vi "Rotation.vi"(8 "C Y":dbl=540.0, 9 "C X":dbl=960.0, 10 "Y":dbl, 11 "X":dbl) -> (1 "Rot Y":dbl, 2 "Rot X":dbl)   [LabVIEW 2020, in "obs-scratch.lvlib"]
uses:
  obs-scratch.lvlib
panel:
  in  "Rotation":dbl(slide) scale=-180.0..180.0
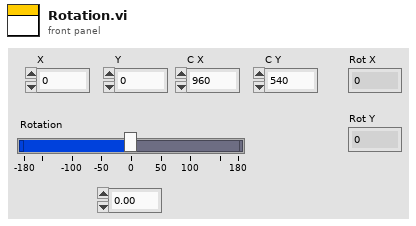
[diagram p1: front panel]
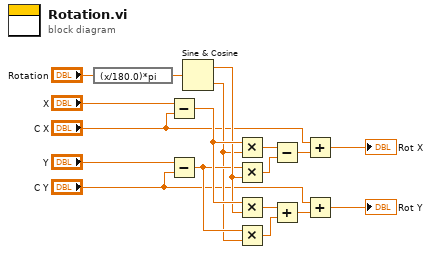
[diagram p0: block diagram]
diagram:
  n1 = expression code="(x/180.0)*pi" ("degrees to radians")("Rotation") -> (w7:dbl)
  n2 = Subtract(x="X", y="C X") -> (x-y=w13:dbl)
  n3 = Subtract(x="Y", y="C Y") -> (x-y=w11:dbl)
  n4 = Sine & Cosine(0:w7) -> (1:w12:dbl, 2:w10:dbl)
  n5 = Multiply(x=w13, y=w10) -> (x*y=w15:dbl)
  n6 = Multiply(x=w11, y=w12) -> (x*y=w14:dbl)
  n7 = Multiply(x=w13, y=w12) -> (x*y=w9:dbl)
  n8 = Multiply(x=w11, y=w10) -> (x*y=w8:dbl)
  n9 = Subtract(x=w15, y=w14) -> (x-y=w6:dbl)
  n10 = Add(x=w9, y=w8) -> (x+y=w4:dbl)
  n11 = Add(x="C X", y=w6) -> (x+y=→"Rot X":dbl)
  n12 = Add(x="C Y", y=w4) -> (x+y=→"Rot Y":dbl)
